vi "Teleop.vi"(10 "Match Info":T1={"Autonomous Elapsed Seconds"=0.0, "TeleOp Elapsed Seconds"=0.0, "Disabled Elapsed Seconds"=0.0, "Visited Autonomous"=FALSE, "Visited TeleOp"=FALSE, "Visited Disabled"=FALSE, "Autonomous Settings"={"Autonomous Style"=enum."Independent", "VI Refnum"=refnum}}, 11 "Call Context":T2) -> ()   [LabVIEW 2015]
doc: "This VI is called for each TeleOp packet received from the DS where the robot is not disabled. It is often used to read from the joysticks and update I/O or to update setpoints for timed control loops. It should complete and return within 20 milliseconds or it may miss DS packets."
uses:
  <vilib>/Rock Robotics/WPI/DriverStation/WPI_DriverStationDerivedRobotMode.ctl
  <vilib>/Rock Robotics/WPI/DriverStation/WPI_DriverStationMatch Info.ctl
  <vilib>/Rock Robotics/WPI/Utilities/WPI_GetSetVariantRefNum.vi
  <vilib>/Rock Robotics/Network Tables/NT Read Boolean.vi
  <vilib>/Rock Robotics/Network Tables/NT Read Number.vi
panel:
  out "Sample Slider 0":dbl(slide) scale=0.0..5.0
  out "Sample Boolean 1":bool
  out "Sample Boolean 0":bool
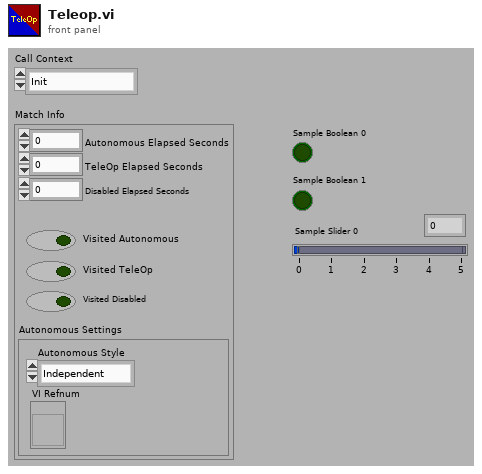
[diagram p1: front panel]
types:
  T1 = typedef "WPI_DriverStationMatch Info.ctl" = cluster{"Autonomous Elapsed Seconds":dbl, "TeleOp Elapsed Seconds":dbl, "Disabled Elapsed Seconds":dbl, "Visited Autonomous":bool, "Visited TeleOp":bool, "Visited Disabled":bool, "Autonomous Settings":cluster{"Autonomous Style":enum16{"Iterative", "Independent"}, "VI Refnum":refnum<vi>}}
  T2 = typedef "WPI_DriverStationDerivedRobotMode.ctl" = enum16{"Init", "Execute", "Stop"}
  T3 = typedef "WPI_JoystickDevRef.ctl" = cluster{"Device":T4}
  T4 = typedef "WPI_JoystickDeviceEnum.ctl" = enum16{"USB 0", "USB 1", "USB 2", "USB 3", "USB 4", "USB 5"}
  T5 = typedef "WPI_MotorControlDeviceRef.ctl" = cluster{"DeviceStatus":errorcluster, "Type":T6, "PWM":cluster{"PWM Channel":T7, "DeadBand":T8}, "CAN":cluster{"Device Number":u8, "Control Mode":T9, "Semaphore":T10, "Max Vout":dbl, "TalonSRX Control Mode":T11}, "Invert":bool}
  T6 = typedef "WPI_MotorControlType.ctl" = enum16{"PWM", "CAN", "CANTalonSRX"}
  T7 = typedef "FPGA_DIOPWMChannel.ctl" = enum8{"PWM 0", "PWM 1", "PWM 2", "PWM 3", "PWM 4", "PWM 5", "PWM 6", "PWM 7", "PWM 8", "PWM 9", "PWM MXP 0", "PWM MXP 1", "PWM MXP 2", "PWM MXP 3", "PWM MXP 4", "PWM MXP 5", "PWM MXP 6", "PWM MXP 7", "PWM MXP 8", "PWM MXP 9", "Invalid"}
  T8 = typedef "WPI_PWMDeadband.ctl" = cluster{"Name":string, "maxPositivePwm":i32, "minPositivePwm":i32, "centerPwm":i32, "maxNegativePwm":i32, "minNegativePwm":i32, "angularRange":u16}
  T9 = typedef "WPI_CANJaguar_ControlMode.ctl" = enum8{"Percent VBus", "Current", "Speed", "Position", "Voltage"}
  T10 = typedef "Semaphore RefNum" = refnum<k1>
  T11 = typedef "WPI_CANTalonSRX_APIControlMode.ctl" = enum8{"Percent VBus", "Speed", "Position", "Slave", "Unchanged / Invalid", "Voltage Compensation", "Current", "Motion Profile"}
  T12 = typedef "WPI_ServoDeviceRef.ctl" = cluster{"DeviceStatus":errorcluster, "PWM Channel":T7, "DeadBand":T8}
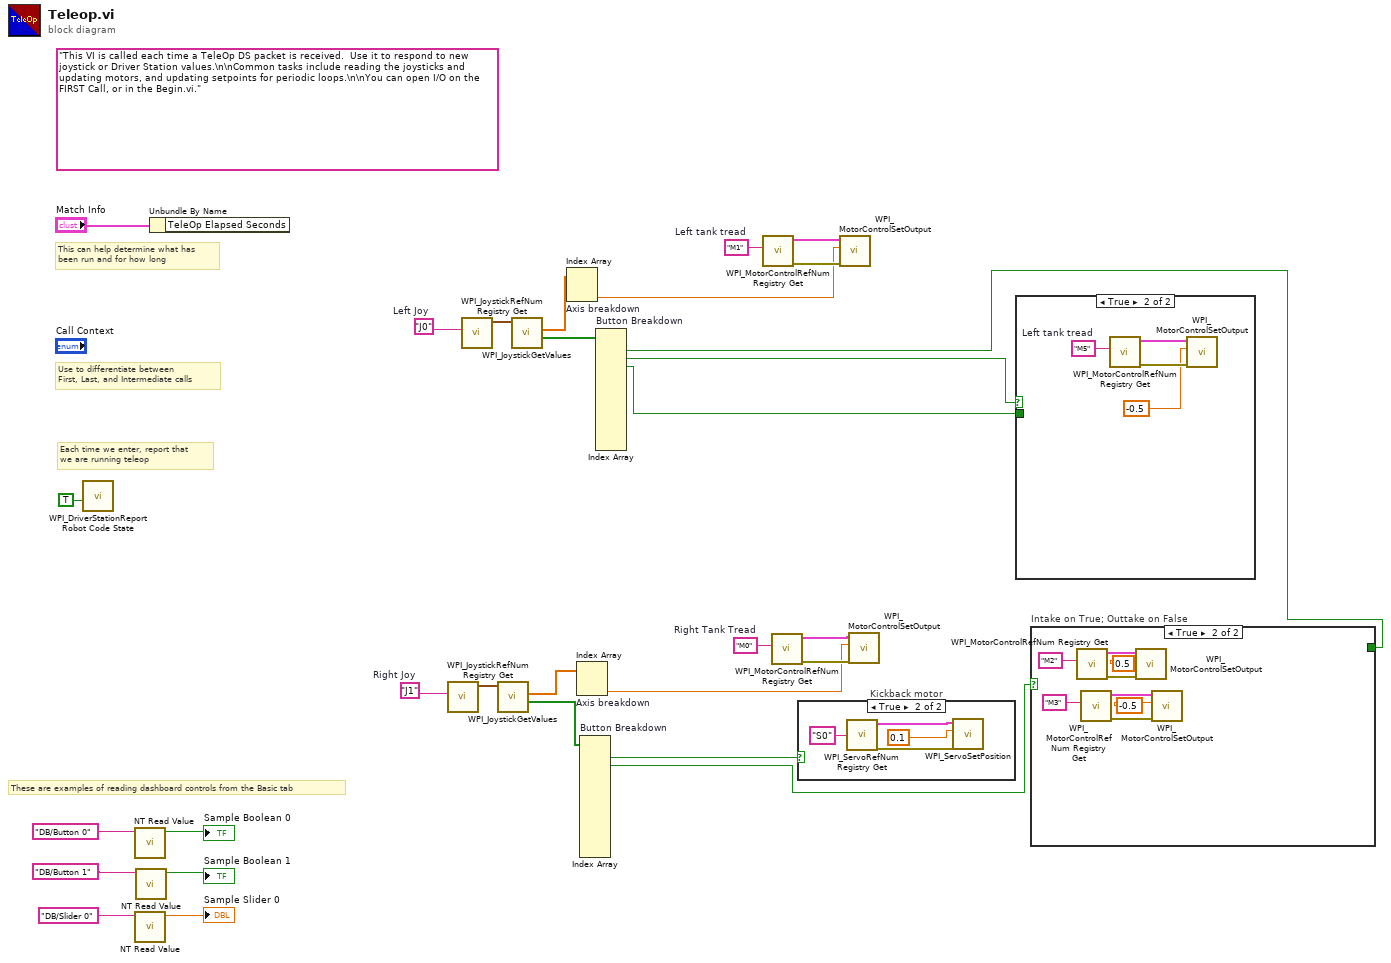
[diagram p0: block diagram]
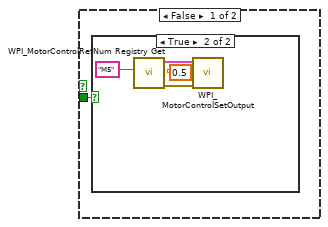
[diagram p2: hidden frame]
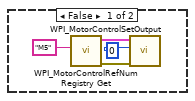
[diagram p3: hidden frame]
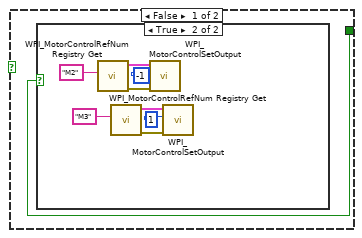
[diagram p4: hidden frame]
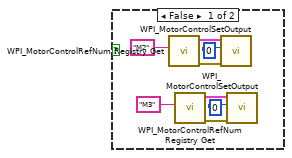
[diagram p5: hidden frame]
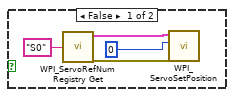
[diagram p6: hidden frame]
diagram:
  w9 = "M0"  # Right Tank Tread
  w11 = "M1"  # Left tank tread
  w17 = "J1"  # Right Joy
  (unwired) "This VI is called each time a TeleOp DS packet is received.  Use it to respond to new joystick or Driver Station values.\n\nCommon tasks include reading the joysticks and updating motors, and updating setpoints for periodic loops.\n\nYou can open I/O on the FIRST Call, or in the Begin.vi."
  w28 = "J0"  # Left Joy
  # "These are examples of reading dashboard controls from the Basic tab"
  # "Each time we enter, report that\nwe are running teleop"
  # "Use to differentiate between\nFirst, Last, and Intermediate calls"
  # "This can help determine what has\nbeen run and for how long"
  n1 = call <vilib>:"WPI_DriverStationReport Robot Code State.vi"("TeleOp"=TRUE ("Autonomous")) -> ()  [unwired: 10 in, 1 out]
  n2 = call-poly <vilib>:"NT Read Value.vi"("Name"="DB/Button 0" ("refnum name")) -> ("Boolean"=→"Sample Boolean 0":bool)  [unwired: 9 in, 1 out]
  n3 = call-poly <vilib>:"NT Read Value.vi"("Name"="DB/Slider 0" ("refnum name")) -> ("Numeric"=→"Sample Slider 0":dbl)  [unwired: 9 in, 1 out]
  n4 = call-poly <vilib>:"NT Read Value.vi"("Name"="DB/Button 1" ("refnum name")) -> ("Boolean"=→"Sample Boolean 1":bool)  [unwired: 9 in, 1 out]
  n5 = Unbundle By Name("Match Info") -> ()  [unwired: 1 out]
  n6 = call <vilib>:"WPI_JoystickRefNum Registry Get.vi"("refnum name"=w17) -> ("JoystickDevRef"=w16:T3)  [unwired: 1 in, 9 out]
  n7 = call <vilib>:"WPI_JoystickRefNum Registry Get.vi"("refnum name"=w28) -> ("JoystickDevRef"=w27:T3)  [unwired: 1 in, 9 out]
  n8 = call <vilib>:"WPI_JoystickGetValues.vi"("JoystickDevRef"=w16) -> ("Buttons"=w14:bool[], "Axes"=w15:dbl[])  [unwired: 6 in, 3 out]
  n9 = call <vilib>:"WPI_JoystickGetValues.vi"("JoystickDevRef"=w27) -> ("Buttons"=w18:bool[], "Axes"=w25:dbl[])  [unwired: 6 in, 3 out]
  n10 = Index Array "Axis breakdown"(array=w25) -> (element #2=w2:dbl)  [unwired: 2 in, 1 out]
  n11 = Index Array "Axis breakdown"(array=w15) -> (element #2=w1:dbl)  [unwired: 2 in, 1 out]
  n12 = Index Array "Button Breakdown"(array=w14) -> (element #1=w13:bool, element #2=w6:bool)  [unwired: 13 in, 11 out]
  n13 = Index Array "Button Breakdown"(array=w18) -> (element #1=w5:bool, element #2=w4:bool, element #3=w3:bool)  [unwired: 13 in, 10 out]
  n14 = call <vilib>:"WPI_MotorControlRefNum Registry Get.vi"("refnum name"=w11) -> ("error out"=w10:errorcluster, "MotorControlDevRef"=w12:T5)  [unwired: 9 in]
  n15 = call <vilib>:"WPI_MotorControlRefNum Registry Get.vi"("refnum name"=w9) -> ("error out"=w8:errorcluster, "MotorControlDevRef"=w7:T5)  [unwired: 9 in]
  n16 = case "Kickback motor" shown="True" w13 {
    frame False {
      n17 = call <vilib>:"WPI_ServoRefNum Registry Get.vi"("refnum name"="S0") -> ("error out"=w31:errorcluster, "ServoDeviceRef"=w32:T12)  [unwired: 9 in]
      n18 = call <vilib>:"WPI_ServoSetPosition.vi"("error in (no error)"=w31, "Position"=0, "ServoDeviceRef"=w32) -> ()  [unwired: 7 in, 2 out]
    }
    frame True {
      n19 = call <vilib>:"WPI_ServoRefNum Registry Get.vi"("refnum name"="S0") -> ("error out"=w35:errorcluster, "ServoDeviceRef"=w36:T12)  [unwired: 9 in]
      n20 = call <vilib>:"WPI_ServoSetPosition.vi"("error in (no error)"=w35, "Position"=0.1, "ServoDeviceRef"=w36) -> ()  [unwired: 7 in, 2 out]
    }
  }
  n21 = call <vilib>:"WPI_MotorControlSetOutput.vi"("error in (no error)"=w10, "Output"=w2, "MotorControlDevRef"=w12) -> ()  [unwired: 6 in, 3 out]
  n22 = call <vilib>:"WPI_MotorControlSetOutput.vi"("error in (no error)"=w8, "Output"=w1, "MotorControlDevRef"=w7) -> ()  [unwired: 6 in, 3 out]
  n23 = case shown="True" w4 {
    tunnel: w3 -> [w38 _]
    frame False {
      n24 = case "Intake on True; Outtake on False" shown="True" w38 {
        frame False {
          n25 = call <vilib>:"WPI_MotorControlRefNum Registry Get.vi"("refnum name"="M5") -> ("error out"=w40:errorcluster, "MotorControlDevRef"=w41:T5)  [unwired: 9 in]
          n26 = call <vilib>:"WPI_MotorControlSetOutput.vi"("error in (no error)"=w40, "Output"=0, "MotorControlDevRef"=w41) -> ()  [unwired: 6 in, 3 out]
        }
        frame True {
          n27 = call <vilib>:"WPI_MotorControlRefNum Registry Get.vi"("refnum name"="M5") -> ("error out"=w44:errorcluster, "MotorControlDevRef"=w45:T5)  [unwired: 9 in]
          n28 = call <vilib>:"WPI_MotorControlSetOutput.vi"("error in (no error)"=w44, "Output"=0.5, "MotorControlDevRef"=w45) -> ()  [unwired: 6 in, 3 out]
        }
      }
    }
    frame True {
      w49 = "M5"  # Left tank tread
      n29 = call <vilib>:"WPI_MotorControlRefNum Registry Get.vi"("refnum name"=w49) -> ("error out"=w48:errorcluster, "MotorControlDevRef"=w50:T5)  [unwired: 9 in]
      n30 = call <vilib>:"WPI_MotorControlSetOutput.vi"("error in (no error)"=w48, "Output"=-0.5, "MotorControlDevRef"=w50) -> ()  [unwired: 6 in, 3 out]
    }
  }
  n31 = case "Intake on True; Outtake on False" shown="True" w6 {
    tunnel: w5 -> [w51 _]
    frame False {
      n32 = case shown="True" w51 {
        frame False {
          n33 = call <vilib>:"WPI_MotorControlRefNum Registry Get.vi"("refnum name"="M2") -> ("error out"=w57:errorcluster, "MotorControlDevRef"=w58:T5)  [unwired: 9 in]
          n34 = call <vilib>:"WPI_MotorControlRefNum Registry Get.vi"("refnum name"="M3") -> ("error out"=w53:errorcluster, "MotorControlDevRef"=w54:T5)  [unwired: 9 in]
          n35 = call <vilib>:"WPI_MotorControlSetOutput.vi"("error in (no error)"=w57, "Output"=0, "MotorControlDevRef"=w58) -> ()  [unwired: 6 in, 3 out]
          n36 = call <vilib>:"WPI_MotorControlSetOutput.vi"("error in (no error)"=w53, "Output"=0, "MotorControlDevRef"=w54) -> ()  [unwired: 6 in, 3 out]
        }
        frame True {
          n37 = call <vilib>:"WPI_MotorControlRefNum Registry Get.vi"("refnum name"="M2") -> ("error out"=w65:errorcluster, "MotorControlDevRef"=w66:T5)  [unwired: 9 in]
          n38 = call <vilib>:"WPI_MotorControlRefNum Registry Get.vi"("refnum name"="M3") -> ("error out"=w61:errorcluster, "MotorControlDevRef"=w62:T5)  [unwired: 9 in]
          n39 = call <vilib>:"WPI_MotorControlSetOutput.vi"("error in (no error)"=w65, "Output"=-1, "MotorControlDevRef"=w66) -> ()  [unwired: 6 in, 3 out]
          n40 = call <vilib>:"WPI_MotorControlSetOutput.vi"("error in (no error)"=w61, "Output"=1, "MotorControlDevRef"=w62) -> ()  [unwired: 6 in, 3 out]
        }
      }
    }
    frame True {
      n41 = call <vilib>:"WPI_MotorControlRefNum Registry Get.vi"("refnum name"="M2") -> ("error out"=w73:errorcluster, "MotorControlDevRef"=w74:T5)  [unwired: 9 in]
      n42 = call <vilib>:"WPI_MotorControlRefNum Registry Get.vi"("refnum name"="M3") -> ("error out"=w69:errorcluster, "MotorControlDevRef"=w70:T5)  [unwired: 9 in]
      n43 = call <vilib>:"WPI_MotorControlSetOutput.vi"("error in (no error)"=w73, "Output"=0.5, "MotorControlDevRef"=w74) -> ()  [unwired: 6 in, 3 out]
      n44 = call <vilib>:"WPI_MotorControlSetOutput.vi"("error in (no error)"=w69, "Output"=-0.5, "MotorControlDevRef"=w70) -> ()  [unwired: 6 in, 3 out]
    }
  }
